vi "Get_4275_Configuration.vi"(8 "error in":errorcluster) -> (0 "error out":errorcluster, 2 "Keystate":string)   [LabVIEW 2020]
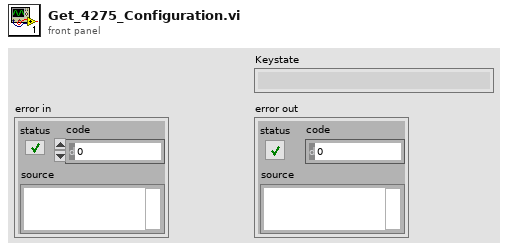
[diagram p1: front panel]
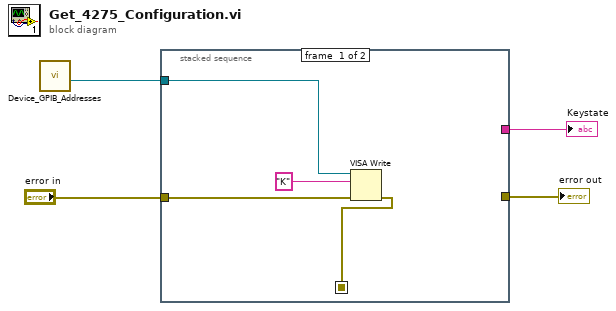
[diagram p0: block diagram]
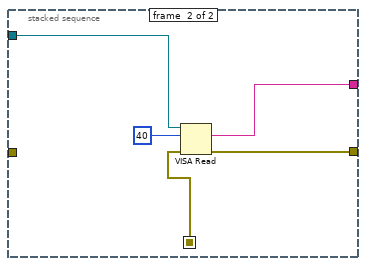
[diagram p2: hidden frame]
diagram:
  n1 = call "Device_GPIB_Addresses.vi"() -> ("HP 4275A Address"=w1:refnum<visa-resource-name>)  [unwired: 9 in, 2 out]
  n2 = stacked-sequence {
    seq-local: [w5 _] -> [_ w11]
    tunnel: "error in" -> [w6 _]
    tunnel: [_ w9] -> w3
    tunnel: [_ w10] -> w2
    tunnel: w1 -> [w8 w13]
    frame #0 {
      n3 = VISA Write(VISA resource name=w8, write buffer="K" ("multi-line string"), error in (no error)=w6) -> (error out=w5:errorcluster)  [unwired: 2 out]
    }
    frame #1 {
      n4 = VISA Read(VISA resource name=w13, byte count=40, error in (no error)=w11) -> (read buffer=w9:string, error out=w10:errorcluster)  [unwired: 2 out]
    }
  }
  "Keystate" <- w3
  "error out" <- w2
